vi "TempToPicWithScale.vi"(0 "Image with Scale":T1(plugin-control), 1 "Bottom prost.":i32, 2 "rozdzielczość obrazu pomniejszona o 30px":i32, 3 "error in (no error)":errorcluster, 4 "Temperatury (wybrany kanał)":dbl[](array[numeric])) -> (5 "Image Out":T1(plugin-control), 6 "step dla 1stC":dbl, 7 "error out":errorcluster)   [LabVIEW 2009]
uses:
  <vilib>/vision/NI_Vision_Development_Module.lvlib
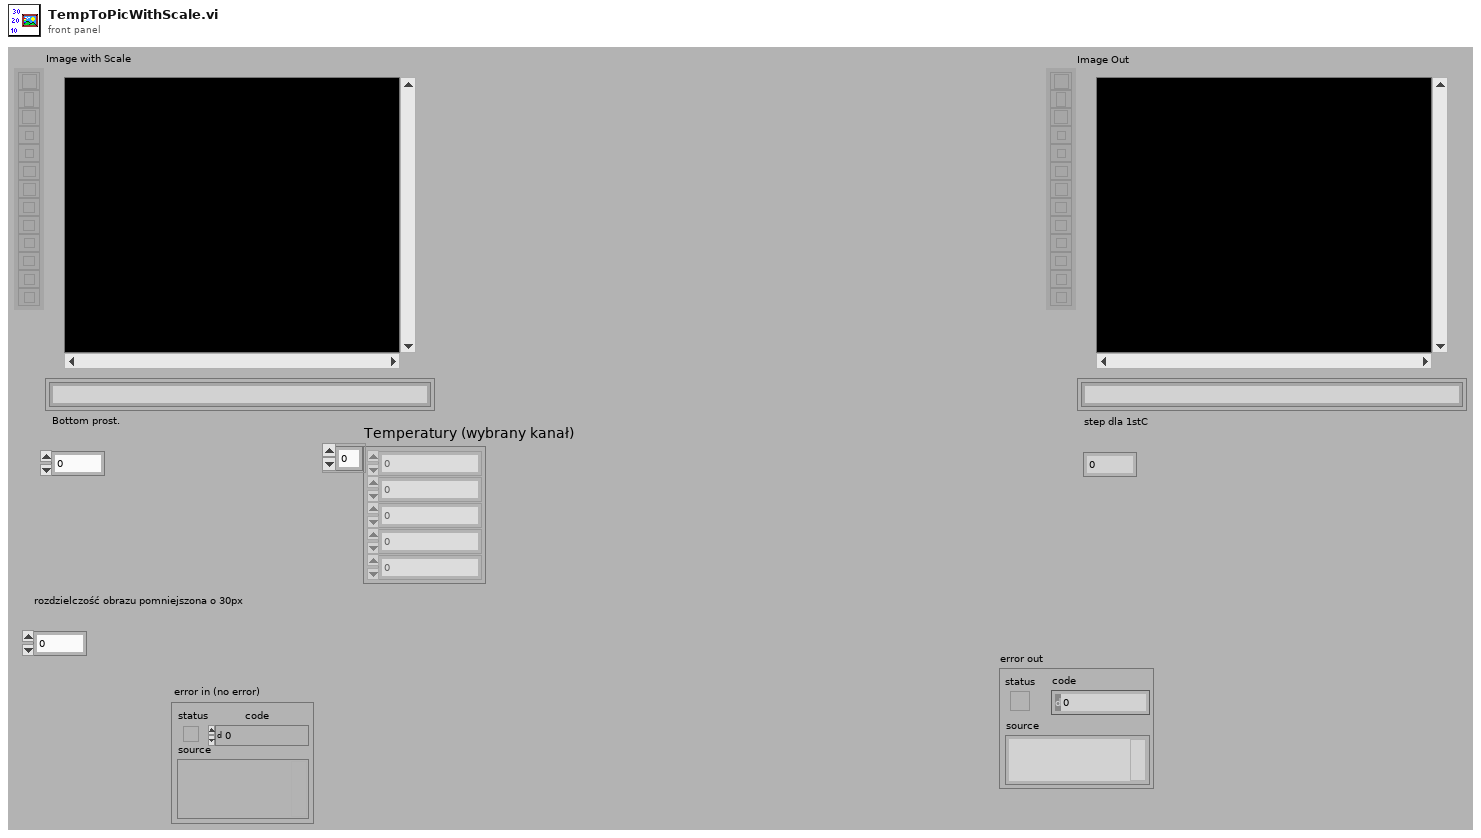
[diagram p1: front panel]
types:
  T1 = typedef "IMAQ Image.ctl" = refnum<image>
  T2 = cluster{"Desired Font (Application)":enum16{"User-specified Font", "Application Font", "System Font", "Dialog Font"}, "[User-specified Font]":cluster{"Font Name":string, "Size":i16, "Strikeout?":bool, "Italic?":bool, "Underline?":bool, "Outline?":bool, "Shadow?":bool, "Bold?":bool, "Rotation Angle":dbl}, "Horizontal Alignment":i16, "Vertical Alignment":i16}
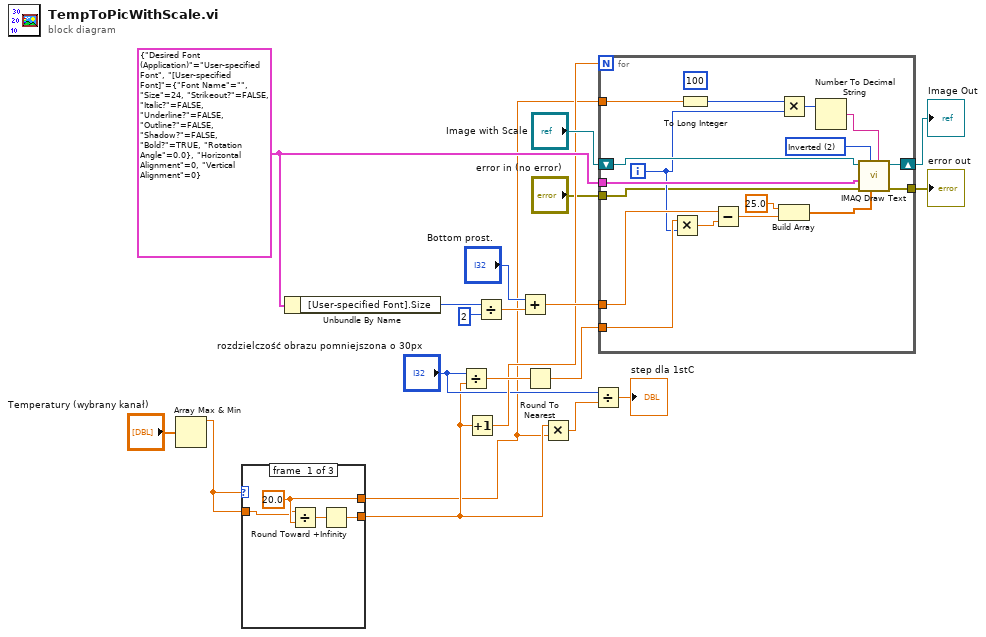
[diagram p0: block diagram]
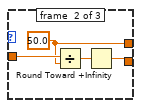
[diagram p2: hidden frame]
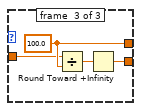
[diagram p3: hidden frame]
diagram:
  w14 = T2 {"Desired Font (Application)"=enum."User-specified Font", "[User-specified Font]"={"Font Name"="", "Size"=24, "Strikeout?"=FALSE, "Italic?"=FALSE, "Underline?"=FALSE, "Outline?"=FALSE, "Shadow?"=FALSE, "Bold?"=TRUE, "Rotation Angle"=0.0}, "Horizontal Alignment"=0, "Vertical Alignment"=0} ("Font, Size & Style")
  n1 = Array Max & Min(array="Temperatury (wybrany kanał)") -> (max value=w2:dbl)  [unwired: 3 out]
  n2 = case shown="..200" w2 {
    tunnel: [w23 w27 w31] -> w3
    tunnel: [w22 w25 w30] -> w1
    tunnel: w2 -> [w21 w26 w29]
    frame #0 {
      w22 = 20.0 ("y")
      n3 = Divide(x=w21, y=w22) -> (x/y=w24:dbl)
      n4 = Round Toward +Infinity(x=w24) -> (ceil(x): smallest int >= x=w23:dbl)
    }
    frame #1 {
      w25 = 50.0 ("y")
      n5 = Divide(x=w26, y=w25) -> (x/y=w28:dbl)
      n6 = Round Toward +Infinity(x=w28) -> (ceil(x): smallest int >= x=w27:dbl)
    }
    frame #2 {
      w30 = 100.0 ("y")
      n7 = Divide(x=w29, y=w30) -> (x/y=w32:dbl)
      n8 = Round Toward +Infinity(x=w32) -> (ceil(x): smallest int >= x=w31:dbl)
    }
  }
  n9 = Unbundle By Name(w14) -> ("[User-specified Font].Size"=w13:i16)
  n10 = Divide(x="rozdzielczość obrazu pomniejszona o 30px", y=w3) -> (x/y=w19:dbl)
  n11 = Increment(x=w3) -> (x+1=w9:dbl)
  n12 = Divide(x=w13, y=i16 2) -> (x/y=w10:dbl)
  n13 = Add(x="Bottom prost.", y=w10) -> (x+y=w11:dbl)
  n14 = Round To Nearest(number=w19) -> (nearest integer value=w15:dbl)
  n15 = Multiply(x=w3, y=w1) -> (x*y=w7:dbl)
  n16 = Divide(x="rozdzielczość obrazu pomniejszona o 30px", y=w7) -> (x/y=→"step dla 1stC":dbl)
  n17 = for {
    N: w9 -> [_]
    tunnel: w15 -> [w45]
    shift-right: [w47] -> w16
    shift-left: "Image with Scale" -> [w49]
    tunnel: w11 -> [w43]
    tunnel: w14 -> [w40]
    tunnel: "error in (no error)" -> [w36]
    tunnel: [w35] -> w4
    tunnel: w1 -> [w34]
    i -> [w38]
    (unwired) 100 ("x")
    w48 = 2 items=["White", "Black", "Inverted", "Black on White", "White on Black"] ("Color")
    n18 = Multiply(x=w45, y=w38) -> (x*y=w44:dbl)
    n19 = To Long Integer(number=w34) -> (32bit integer=w33:i32)
    n20 = Subtract(x=w43, y=w44) -> (x-y=w42:dbl)
    n21 = Multiply(x=w33, y=w38) -> (x*y=w39:i32)
    n22 = Build Array(25.0 ("element"), w42) -> (w41:dbl[])
    n23 = Number To Decimal String(number=w39) -> (decimal integer string=w37:string)  [unwired: 1 in]
    n24 = call "IMAQ Draw Text"("String"=w37, "Insertion Point"=w41, "Color"=w48, "error in (no error)"=w36, "Font, Size & Style"=w40, "Image Src"=w49) -> ("error out"=w35:errorcluster, "Image Dst Out"=w47:T1)  [unwired: 2 in, 2 out]
  }
  "Image Out" <- w16
  "error out" <- w4
